vi "Boolean_Change.vi"(2 "Error In":errorcluster, 3 "Input":bool) -> (0 "Error Out":errorcluster, 1 "Output":bool)   [LabVIEW 2019]
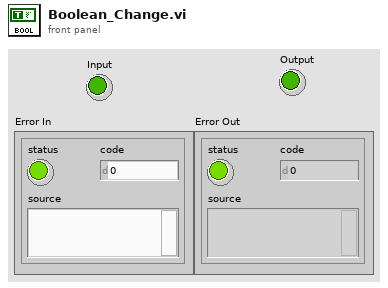
[diagram p1: front panel]
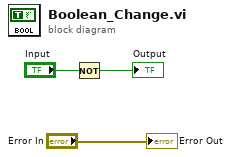
[diagram p0: block diagram]
diagram:
  n1 = Not(x="Input") -> (.not. x?=→"Output":bool)
  "Error Out" <- "Error In"
